vi "Test_AddUnnamedTopic_NoOpReturnError.vi"(8 "error in (no error)":errorcluster, 11 "TestCase in":refnum<class "TestTopicLookupTable.lvclass">) -> (0 "error out":errorcluster, 3 "TestCase out":refnum<class "TestTopicLookupTable.lvclass">)   [LabVIEW 2017, in "TestTopicLookupTable.lvclass"]
uses:
  TestTopicLookupTable.lvclass
  <vilib>/ActorFramework/Message Queue/Message Queue.lvclass/Message Queue.ctl
  Topic/Topic.lvclass/Topic.ctl
  TopicLookupTable/TopicLookupTable.lvclass/TopicLookupTable.ctl
  Topic/Read Topic Info.vi
  <vilib>/ActorFramework/Actor/Read Self Enqueuer.vi
  <vilib>/ActorFramework/Message Enqueuer/Init from Existing Queue.vi
  gpm_packages/@cs/variant/Source/Format Type String.vi
  <vilib>/ActorFramework/Message Enqueuer/Message Enqueuer.lvclass
  <vilib>/addons/_JKI Toolkits/VI Tester/TestCase.llb/TestCase.lvclass
  TopicLookupTable/TopicLookupTable.lvclass
  Topic/Topic.lvclass
  <vilib>/ActorFramework/Message Queue/Message Queue.lvclass
  C:/Program Files (x86)/National Instruments/LabVIEW 2017/vi.lib/addons/_JKI Toolkits/VI Tester/TestCase.llb/TestCase.lvclass
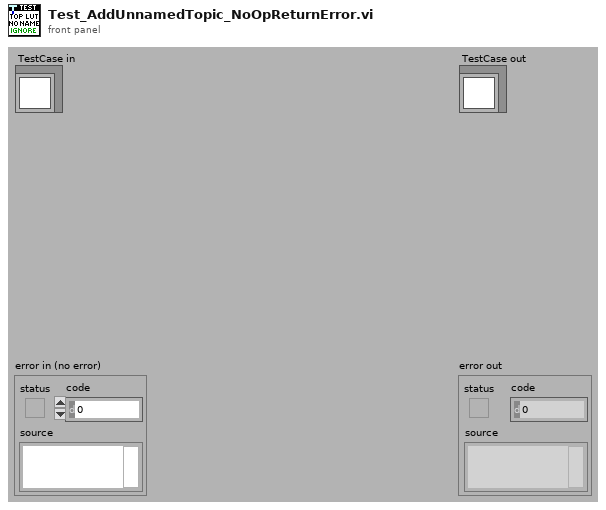
[diagram p1: front panel]
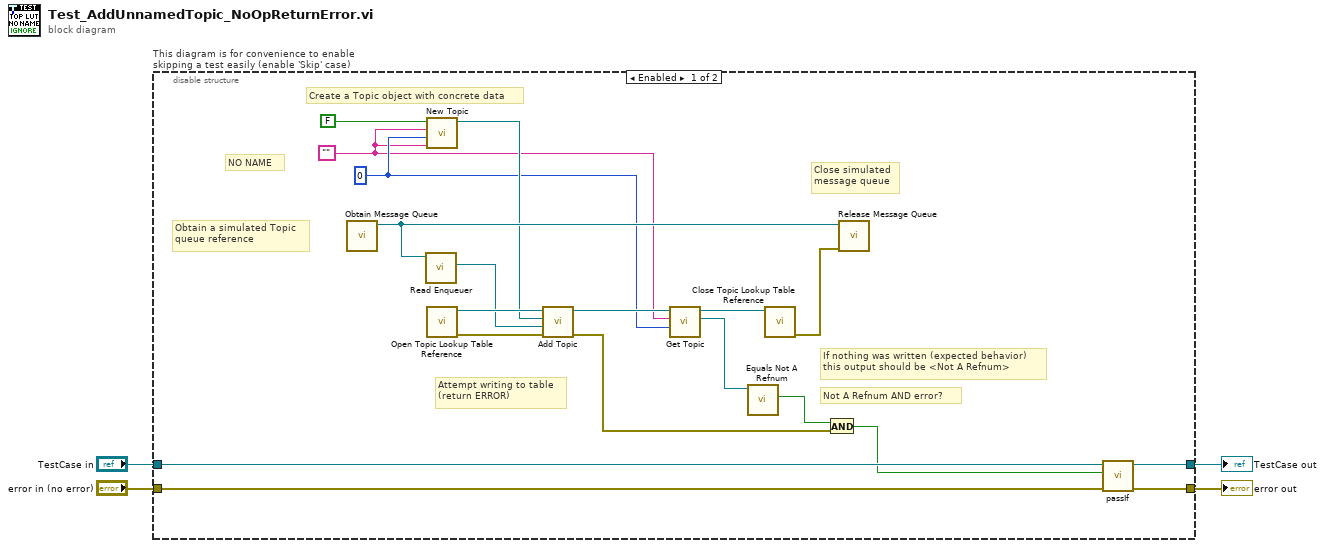
[diagram p0: block diagram]
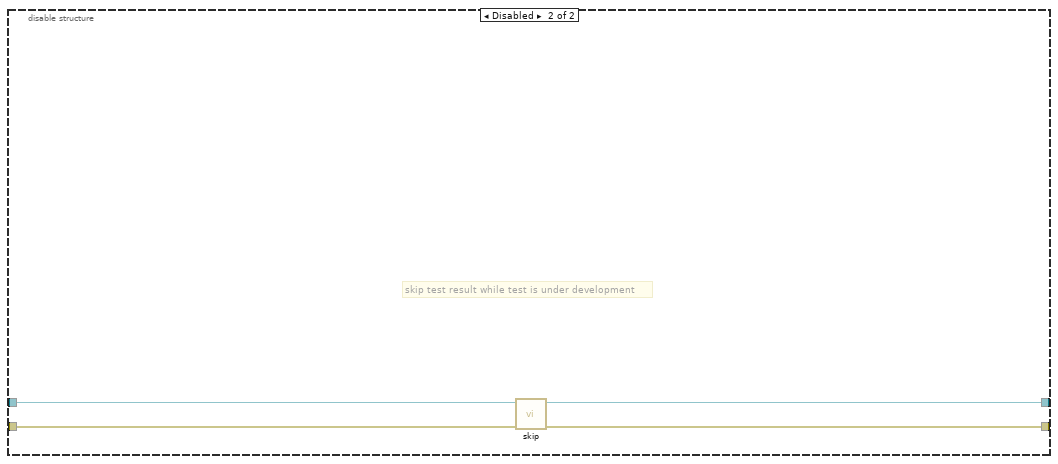
[diagram p2: hidden frame]
diagram:
  n1 = disable-structure "This diagram is for convenience to enable skipping a test easily (enable 'Skip' case)" shown="Enabled" {
    disable-tunnel: "TestCase in" -> [w23 w27]
    disable-tunnel: [w22 w25] -> w1
    disable-tunnel: [w21 w26] -> w3
    disable-tunnel: "error in (no error)" -> [w20 w24]
    frame Enabled {
      w10 = 0
      w5 = "" ("Name")
      # "Not A Refnum AND error?"
      # "If nothing was written (expected behavior)\nthis output should be <Not A Refnum>"
      # "NO NAME"
      # "Create a Topic object with concrete data"
      # "Attempt writing to table\n(return ERROR)"
      # "Close simulated\nmessage queue"
      # "Obtain a simulated Topic\nqueue reference"
      n2 = call <vilib>:"Obtain Message Queue.vi"() -> ("Message Queue"=w14:refnum<class "Message Queue.lvclass">)  [unwired: 10 in, 1 out]
      n3 = call <vilib>:"Read Enqueuer.vi"("Message Queue"=w14) -> ("Message Enqueuer"=w16:refnum<class "Message Enqueuer.lvclass">)  [unwired: 10 in]
      n4 = call "New Topic.vi"("Lock Owner ID (\"\" = NOT Locked)"=w5, "New Topic Data"=w10, "Name"=w5, "Use Type Input As Initial Value?"=FALSE) -> ("Topic out"=w12:refnum<class "Topic.lvclass">)  [unwired: 6 in, 1 out]
      n5 = call "Open Topic Lookup Table Reference.vi"() -> ("error out"=w18:errorcluster, "TopicLookupTable Reference"=w19:refnum<data-value>)  [unwired: 10 in]
      n6 = call "Add Topic.vi"("error in (no error)"=w18, "Topic Enqueuer"=w16, "Topic Object"=w12, "TopicLookupTable"=w19) -> ("error out"=w7:errorcluster, "TopicLookupTable"=w17:refnum<data-value>)  [unwired: 5 in, 1 out]
      n7 = call "Get Topic.vi"("Topic Type"=w10, "Topic Name"=w5, "TopicLookupTable"=w17) -> ("Topic Enqueuer"=w9:refnum<class "Message Enqueuer.lvclass">, "TopicLookupTable"=w11:refnum<data-value>)  [unwired: 6 in, 1 out]
      n8 = call <vilib>:"Equals Not A Refnum.vi"("Message Enqueuer"=w9) -> ("Not a refnum?"=w8:bool)  [unwired: 10 in]
      n9 = call "Close Topic Lookup Table Reference.vi"("TopicLookupTable"=w11) -> ("error out"=w15:errorcluster)  [unwired: 10 in]
      n10 = And(x=w8, y=w7) -> (x .and. y?=w6:bool)
      n11 = call <vilib>:"Release Message Queue.vi"("error in (no error)"=w15, "Message Queue"=w14) -> ()  [unwired: 8 in, 2 out]
      n12 = call-dynamic "passIf.vi"("error in (no error)"=w20, "pass"=w6, "TestCase in"=w23) -> ("error out"=w21:errorcluster, "TestCase out"=w22:refnum<class "TestTopicLookupTable.lvclass">)  [unwired: 7 in]
    }
    frame Disabled {
      # "skip test result while test is under development"
      n13 = call <vilib>:"skip.vi"("error in (no error)"=w24, "TestCase in"=w27) -> ("error out"=w26:errorcluster, "TestCase out"=w25:refnum<class "TestTopicLookupTable.lvclass">)  [unwired: 8 in]
    }
  }
  "error out" <- w3
  "TestCase out" <- w1
